vi "Folder Path to String.vi"(8 "error in":errorcluster, 11 "CD Folder Path":path) -> (0 "error out":errorcluster, 3 "Path as String":string)   [LabVIEW 2026, in "NIVS_CDEW_MetaDataObj.lvclass"]
uses:
  NIVS_CDEW_MetaDataObj.lvclass
  NIVS_CDEW_MetaDataObj.lvclass/NIVS_CDEW_MetaDataObj.ctl
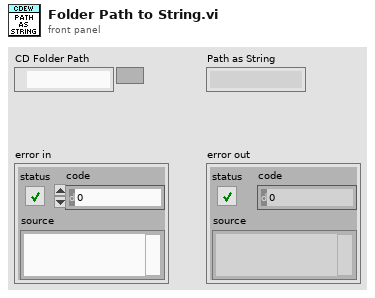
[diagram p1: front panel]
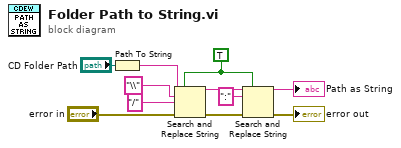
[diagram p0: block diagram]
diagram:
  w5 = TRUE ("replace all? (F)")
  n1 = Path To String(path="CD Folder Path") -> (string=w10:string)
  n2 = Search and Replace String(replace all?=w5, input string=w10, search string="\\", replace string="/" ("replace string (\"\")"), error in="error in") -> (result string=w7:string, error out=w2:errorcluster)  [unwired: 3 in, 2 out]
  n3 = Search and Replace String(replace all?=w5, input string=w7, search string=":", error in=w2) -> (result string=→"Path as String":string, error out=→"error out":errorcluster)  [unwired: 4 in, 2 out]
